vi "ImportCSV.vi"(8 "error in (no error)":errorcluster, 10 "selected path":path, 11 "Node Ref In":T1 format="%.0x") -> (0 "error out":errorcluster)   [LabVIEW 2024, in "Embedded TDMS Logger System Explorer.lvlib"]
doc: "Import the configuration of the Custom Device based on a CSV file. Note: Is legacy code and only maintained for the purposes of non-code users in a specific project set."
uses:
  Embedded TDMS Logger System Explorer.lvlib
  <vilib>/NI VeriStand/Custom Device API/Custom Device Item Ref.ctl
  Shared/File Classes/Meta Data.ctl
  <vilib>/NI VeriStand/Custom Device API/Custom Device Channel.ctl
  <vilib>/NI VeriStand/Custom Device API/Custom Device Channel Type.ctl
  <vilib>/Utility/file.llb/Read Delimited Spreadsheet (string).vi
  Shared/Constants.vi
  <vilib>/NI VeriStand/Custom Device API/Set Item Property (Boolean).vi
  <vilib>/NI VeriStand/Custom Device API/Set Item Property (Variant).vi
  <vilib>/NI VeriStand/Custom Device API/Set Item Property (I32).vi
  <vilib>/NI VeriStand/Custom Device API/Set Item Property (Dependent Node Pointer).vi
  <vilib>/Utility/file.llb/Write Delimited Spreadsheet (string).vi
  NationalInstruments.VeriStand.SystemStorage
  NationalInstruments.VeriStand.SystemDefinitionAPI
  <vilib>/NI VeriStand/Custom Device API/Custom Device API.lvlib
  Shared/Embedded TDMS Logger Shared.lvlib
  <vilib>/NI VeriStand/Custom Device Tools/Custom Device Utility Library/Custom Device Utility Library.lvlib
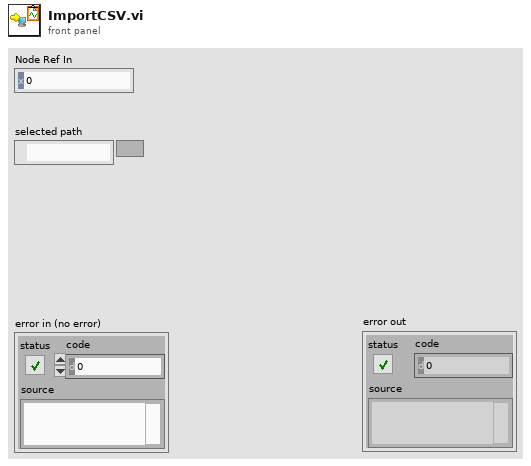
[diagram p1: front panel]
types:
  T1 = typedef "Custom Device API.lvlib/Custom Device Item Ref.ctl" = u64
  T2 = typedef "Custom Device API.lvlib/Custom Device Pointer.ctl" = refnum<k24>
  T3 = typedef "Custom Device API.lvlib/Custom Device Channel.ctl" = cluster{"Type":T4, "Units":string, "Default Value":dbl, "Faultable":bool, "Scalable":bool}
  T4 = typedef "Custom Device API.lvlib/Custom Device Channel Type.ctl" = enum16{"Input", "Output"}
  T5 = typedef "Meta Data.ctl" = cluster{"Key":string, "Value":string}
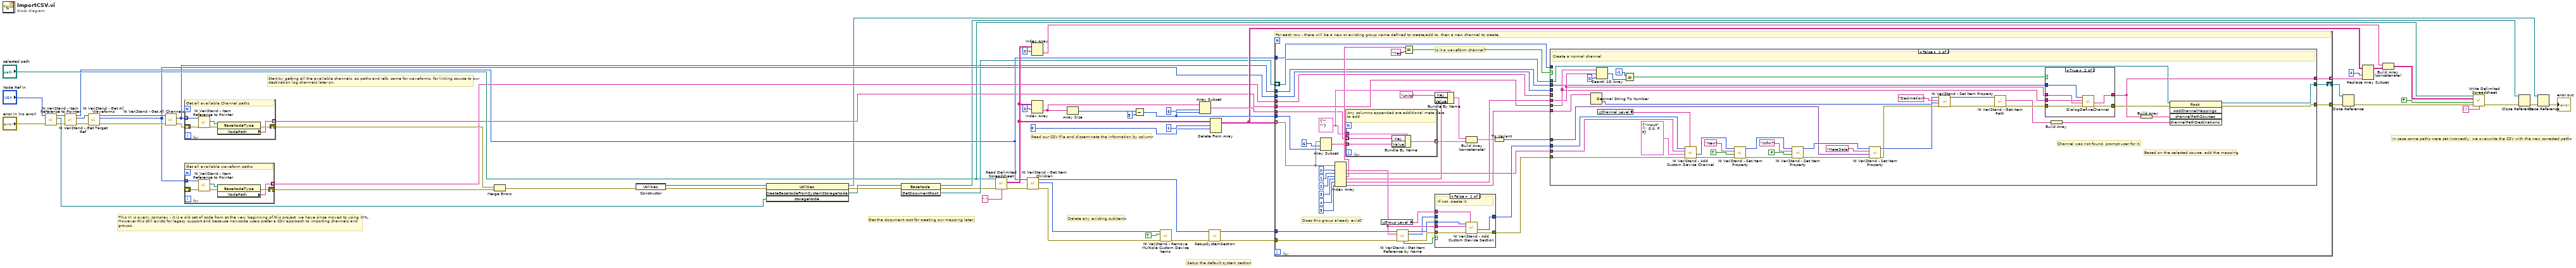
[diagram p0: block diagram]
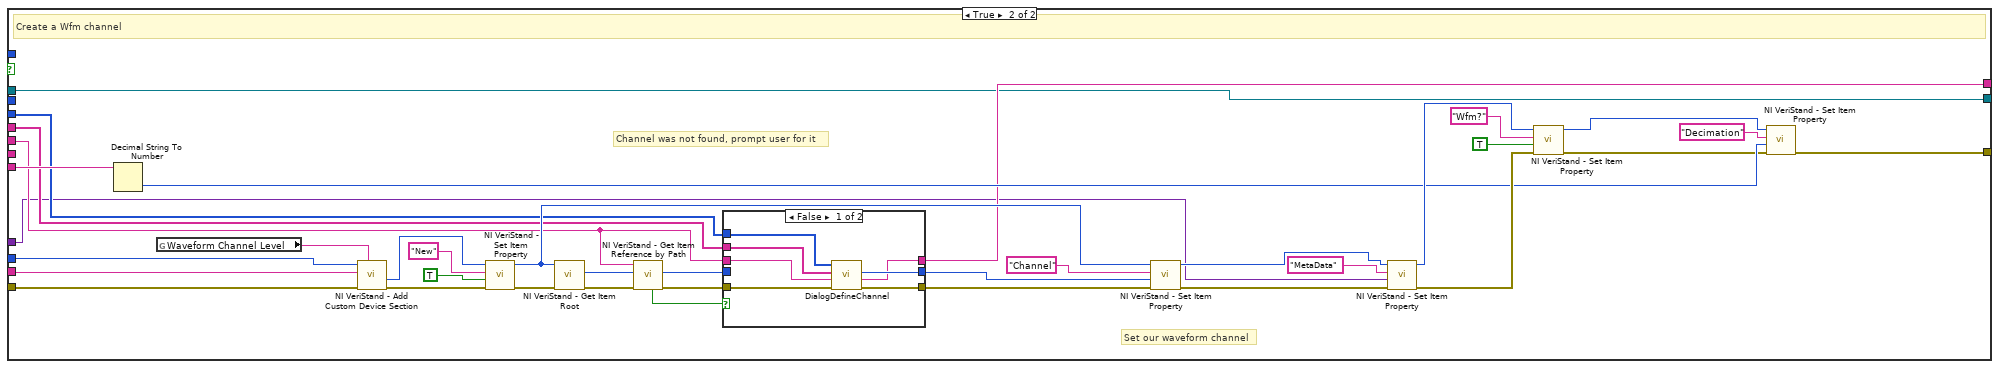
[diagram p3: hidden frame]
diagram:
  # "In case some paths were set incorrectly, we overwrite the CSV with the new corrected paths"
  # "Delete any existing subitems"
  # "Setup the default system section"
  # "Read our CSV file and disseminate the information by column"
  # "Get the document root for creating our mapping later."
  # "Start by getting all the available channels, as paths and refs, same for waveforms, for linking source to our\ndestination log channels later on."
  # "This VI is overly complex - it is a old set of code from at the very beginning of this project, we have since moved to using XML.\nHowever this still exists for legacy support and because non-code users prefer a CSV approach to importing channels and\ngroups."
  n1 = call <vilib>:"NI VeriStand - Item Reference to Pointer.vi"("error in (no error)"="error in (no error)", "Item Ref in"="Node Ref In") -> ("error out"=w18:errorcluster, "Node Pointer"=w23:T2, "Item Ref out"=w17:T1)  [unwired: 6 in, 1 out]
  n2 = call <vilib>:"NI VeriStand - Get Target Ref.vi"("error in"=w18, "Item Ref in"=w17) -> ("error out"=w19:errorcluster, "Target Ref"=w20:T1, "Item Ref out"=w16:T1)  [unwired: 6 in, 1 out]
  n3 = call <vilib>:"NI VeriStand - Get All Waveforms.vi"("error in"=w19, "Section Ref in"=w20) -> ("error out"=w27:errorcluster, "Waveform Refs"=w13:T1[], "Section Ref out"=w28:T1)  [unwired: 6 in, 1 out]
  n4 = call <vilib>:"NI VeriStand - Get All Channels.vi"("error in"=w27, "Section Ref in"=w28) -> ("error out"=w26:errorcluster, "Channel Refs"=w15:T1[])  [unwired: 6 in, 2 out]
  n5 = for {
    tunnel: w15 -> [w67] mode=indexing
    shift-right: [w62] -> w25
    shift-left: w26 -> [w66]
    tunnel: [w63] -> w14 mode=indexing
    # "Get all available Channel paths"
    n6 = call <vilib>:"NI VeriStand - Item Reference to Pointer.vi"("error in (no error)"=w66, "Item Ref in"=w67) -> ("error out"=w65:errorcluster, "Node Pointer"=w64:T2)  [unwired: 6 in, 2 out]
    n7 = property class="BaseNodeType"(reference=w64, error in=w65) -> (error out=w62:errorcluster, "NodePath"=w63:string)  [unwired: 1 out]
  }
  n8 = for {
    tunnel: w13 -> [w71] mode=indexing
    shift-right: [w69] -> w12
    shift-left: _ -> [w70]
    tunnel: [w68] -> w11 mode=indexing
    # "Get all available waveform paths"
    n9 = call <vilib>:"NI VeriStand - Item Reference to Pointer.vi"("error in (no error)"=w70, "Item Ref in"=w71) -> ("error out"=w73:errorcluster, "Node Pointer"=w72:T2)  [unwired: 6 in, 2 out]
    n10 = property class="BaseNodeType"(reference=w72, error in=w73) -> (error out=w69:errorcluster, "NodePath"=w68:string)  [unwired: 1 out]
  }
  n11 = Merge Errors(w25, w12) -> (w24:errorcluster)
  n12 = constructor class="Utilities"(error in=w24) -> (reference out=w32:refnum<k24>, error out=w31:errorcluster)  [unwired: 2 in, 1 out]
  n13 = invoke class="Utilities" method="CreateBaseNodeFromSystemStorageNode"(reference=w32, error in=w31, "storageNode"=w23) -> (reference out=w4:refnum<k24>, error out=w29:errorcluster, "CreateBaseNodeFromSystemStorageNode"=w30:refnum<k24>)  [unwired: 1 in, 1 out]
  n14 = invoke class="BaseNode" method="GetDocumentRoot"(reference=w30, error in=w29) -> (reference out=w5:refnum<k24>, error out=w9:errorcluster, "GetDocumentRoot"=w10:refnum<k24>)  [unwired: 1 in]
  n15 = call-poly <vilib>:"Read Delimited Spreadsheet.vi"("file path (dialog if empty)"="selected path", "error in (no error)"=w9, "delimiter (\\t)"="," ("delimiter (\\t)")) -> ("all rows"=w59:string[][], "error out"=w34:errorcluster)  [unwired: 7 in, 4 out]
  n16 = call <vilib>:"NI VeriStand - Get Item Children.vi"("error in (no error)"=w34, "Item Ref in"=w16) -> ("error out"=w2:errorcluster, "Child Refs"=w3:T1[], "Item Ref out"=w44:T1)  [unwired: 6 in, 1 out]
  n17 = Index Array(array=w59, index (row)=0) -> (element=w49:string[])  [unwired: 1 in]
  n18 = Index Array(array=w59, index (row)=0) -> (element=w55:string[])  [unwired: 1 in]
  n19 = Array Size(array=w55) -> (size(s)=w56:i32)
  n20 = Subtract(x=w56, y=5) -> (x-y=w61:i32)
  n21 = call <vilib>:"NI VeriStand - Remove Multiple Custom Device Items.vi"("error in (no error)"=w2, "Force Delete (F)"=TRUE, "Item Refs in"=w3) -> ("error out"=w45:errorcluster)  [unwired: 7 in, 1 out]
  n22 = Array Subset(array=w55, index=6, length=w61) -> (w60:string[])
  n23 = call "SetupSystemSection.vi"("error in (no error)"=w45, "Node Ptr"=w44) -> ("error out"=w46:errorcluster, "Parent Ref Out"=w47:T1)  [unwired: 4 in, 4 out]
  n24 = Delete From Array(array=w59, length=1, index (row)=0) -> (array with subset deleted=w53:string[][])  [unwired: 1 in, 1 out]
  n25 = for {
    tunnel: w53 -> [w79] mode=indexing
    tunnel: w47 -> [w110]
    tunnel: w16 -> [w95]
    tunnel: w46 -> [w94]
    tunnel: w13 -> [w92]
    tunnel: w11 -> [w91]
    tunnel: w14 -> [w90]
    tunnel: w15 -> [w93]
    tunnel: [w89] -> w38 mode=indexing
    tunnel: [w88] -> w41
    shift-right: [w87] -> w42
    shift-left: w10 -> [w86]
    tunnel: w60 -> [w75]
    tunnel: w61 -> [w78]
    w76 = T5 {"Key"="", "Value"=""} ("Meta Data")
    # "Does this group already exist?"
    # "Is it a waveform channel?"
    # "For each row - there will be a new or existing group name defined to create/add to, then a new channel to create."
    n26 = Array Subset(array=w79, index=6, length=w78) -> (w77:string[])
    n27 = Index Array(array=w79, index #1=0 ("index"), index #2=1 ("index"), index #3=2 ("index"), index #4=3 ("index"), index #5=4 ("index"), index #6=5 ("index")) -> (element #1=w107:string, element #2=w99:string, element #3=w103:string, element #4=w83:string, element #5=w97:string, element #6=w96:string)
    n28 = for {
      tunnel: w77 -> [w118] mode=indexing
      tunnel: w76 -> [w120]
      tunnel: w75 -> [w119] mode=indexing
      tunnel: [w117] -> w74 mode=indexing
      # "Any columns appended are additional meta data to add"
      n29 = Bundle By Name(cluster=w120, "Key"=w119, "Value"=w118) -> (w117:T5)
    }
    n30 = global read "Constants.vi" "Group Level"() -> (w104:string)
    n31 = call <vilib>:"NI VeriStand - Get Item Reference by Name.vi"("error in (no error)"=w94, "Item Name"=w107, "Parent Ref in"=w110) -> ("error out"=w106:errorcluster, "Item Ref"=w105:T1, "Parent Ref out"=w108:T1, "Found"=w109:bool)  [unwired: 5 in]
    n32 = Equal?(x=w103, y="Yes") -> (x = y?=w101:bool)
    n33 = Bundle By Name(cluster=w76, "Key"="Units", "Value"=w83) -> (w80:T5)
    n34 = case shown="False" w109 {
      tunnel: w108 -> [w221 _]
      tunnel: w107 -> [w220 _]
      tunnel: w106 -> [w219 w222]
      tunnel: [w218 w223] -> w100
      tunnel: w105 -> [_ w223]
      tunnel: [w217 w222] -> w98
      tunnel: w104 -> [w216 _]
      frame False {
        # "If not, create it"
        n35 = call <vilib>:"NI VeriStand - Add Custom Device Section.vi"("GUID (Default Section)"=w216, "error in (no error)"=w219, "Section Name"=w220, "Parent Ref in"=w221) -> ("error out"=w217:errorcluster, "Section Ptr"=w218:T1)  [unwired: 4 in, 2 out]
      }
      frame True {
      }
    }
    n36 = Build Array (concatenate)(w80, w74) -> (w82:T5[])
    n37 = To Variant(anything=w82) -> (Variant=w81:variant)
    n38 = case shown="False" w101 {
      tunnel: w100 -> [w148 w193]
      tunnel: w99 -> [w145 w191]
      tunnel: w98 -> [w147 w190]
      tunnel: w97 -> [w130 w179]
      tunnel: w96 -> [w142 w189]
      tunnel: w95 -> [_ _]
      tunnel: w86 -> [w135 w170]
      tunnel: w93 -> [w127 _]
      tunnel: w92 -> [_ w178]
      tunnel: w91 -> [_ w177]
      tunnel: w90 -> [w128 _]
      tunnel: [w125 w172] -> w89
      tunnel: [w123 w171] -> w88
      tunnel: [w122 w170] -> w87
      tunnel: w81 -> [w121 w169]
      frame False {
        # "Channel was not found, prompt user for it."
        # "Based on the selected source, add the mapping"
        # "Create a normal channel"
        n39 = Decimal String To Number(string=w142) -> (number=w143:i32)  [unwired: 2 in, 1 out]
        n40 = Search 1D Array(1D array=w128, element=w130, start index (0)=0) -> (index of element=w133:i32)
        n41 = global read "Constants.vi" "Channel Level"() -> (w146:string)
        n42 = Equal?(x=-1, y=w133) -> (x = y?=w131:bool)
        n43 = call <vilib>:"NI VeriStand - Add Custom Device Channel.vi"("GUID (Default Channel)"=w146, "error in (no error)"=w147, "Channel"=T3 {"Type"=enum."Input", "Units"="", "Default Value"=0.0, "Faultable"=FALSE, "Scalable"=FALSE}, "Channel Name"=w145, "Parent Ref in"=w148) -> ("error out"=w155:errorcluster, "Channel Ref"=w156:T1)  [unwired: 3 in, 2 out]
        n44 = call-poly <vilib>:"NI VeriStand - Set Item Property.vi"("error in (no error)"=w155, "Value"=TRUE, "Property Name"="New", "Item Ref in"=w156) -> ("error out"=w158:errorcluster, "Item Ref out"=w157:T1)  [unwired: 5 in, 1 out]
        n45 = call-poly <vilib>:"NI VeriStand - Set Item Property.vi"("error in (no error)"=w158, "Value"=FALSE, "Property Name"="Wfm?", "Item Ref in"=w157) -> ("error out"=w160:errorcluster, "Item Ref out"=w159:T1)  [unwired: 5 in, 1 out]
        n46 = call-poly <vilib>:"NI VeriStand - Set Item Property.vi"("error in (no error)"=w160, "Value"=w121, "Property Name"="MetaData", "Item Ref in"=w159) -> ("error out"=w140:errorcluster, "Item Ref out"=w141:T1)  [unwired: 5 in, 1 out]
        n47 = call-poly <vilib>:"NI VeriStand - Set Item Property.vi"("error in (no error)"=w140, "Value"=w143, "Property Name"="Decimation", "Item Ref in"=w141) -> ("error out"=w136:errorcluster, "Item Ref out"=w137:T1)  [unwired: 5 in, 1 out]
        n48 = call <vilib>:"NI VeriStand - Get Item Path.vi"("error in (no error)"=w136, "Item Ref in"=w137) -> ("error out"=w126:errorcluster, "Path"=w124:string)  [unwired: 6 in, 2 out]
        n49 = case shown="True" w131 {
          tunnel: [w162 w168] -> w125
          tunnel: w130 -> [w162 w165]
          tunnel: [w161 w167] -> w129
          tunnel: w128 -> [_ w166]
          tunnel: w127 -> [_ w164]
          tunnel: w126 -> [w161 w163]
          frame False {
          }
          frame True {
            n50 = call "DialogDefineChannel.vi"("error in"=w163, "Input String"=w165, "Available Paths"=w166, "Available Refs"=w164) -> ("error out"=w167:errorcluster, "Selected Path"=w168:string)  [unwired: 4 in, 2 out]
          }
        }
        n51 = Build Array(w124) -> (w138:string[])
        n52 = Build Array(w125) -> (w139:string[])
        n53 = invoke class="Root" method="AddChannelMappings"(reference=w135, error in=w129, "channelPathSources"=w139, "channelPathDestinations"=w138) -> (reference out=w122:refnum<k24>, error out=w123:errorcluster)  [unwired: 1 in, 3 out]
      }
      frame True {
        # "Set our waveform channel"
        # "Channel was not found, prompt user for it"
        # "Create a Wfm channel"
        n54 = Decimal String To Number(string=w189) -> (number=w183:i32)  [unwired: 2 in, 1 out]
        n55 = global read "Constants.vi" "Waveform Channel Level"() -> (w192:string)
        n56 = call <vilib>:"NI VeriStand - Add Custom Device Section.vi"("GUID (Default Section)"=w192, "error in (no error)"=w190, "Section Name"=w191, "Parent Ref in"=w193) -> ("error out"=w200:errorcluster, "Section Ptr"=w201:T1)  [unwired: 3 in, 3 out]
        n57 = call-poly <vilib>:"NI VeriStand - Set Item Property.vi"("error in (no error)"=w200, "Value"=TRUE, "Property Name"="New", "Item Ref in"=w201) -> ("error out"=w186:errorcluster, "Item Ref out"=w187:T1)  [unwired: 5 in, 1 out]
        n58 = call <vilib>:"NI VeriStand - Get Item Root.vi"("error in (no error)"=w186, "Item Ref in"=w187) -> ("error out"=w185:errorcluster, "Root Ref out"=w188:T1)  [unwired: 6 in, 2 out]
        n59 = call <vilib>:"NI VeriStand - Get Item Reference by Path.vi"("error in (no error)"=w185, "Root Ref"=w188, "Item Path in"=w179) -> ("error out"=w176:errorcluster, "Item Ref"=w173:T1, "Found"=w184:bool)  [unwired: 5 in, 1 out]
        n60 = case shown="False" w184 {
          tunnel: w179 -> [w212 w213]
          tunnel: w178 -> [w210 _]
          tunnel: w177 -> [w211 _]
          tunnel: w176 -> [w207 w214]
          tunnel: [w208 w214] -> w175
          tunnel: [w209 w215] -> w174
          tunnel: w173 -> [_ w215]
          tunnel: [w206 w213] -> w172
          frame False {
            n61 = call "DialogDefineChannel.vi"("error in"=w207, "Input String"=w212, "Available Paths"=w211, "Available Refs"=w210) -> ("error out"=w208:errorcluster, "Selected Path"=w206:string, "Selected Ref"=w209:T1)  [unwired: 4 in, 1 out]
          }
          frame True {
          }
        }
        n62 = call-poly <vilib>:"NI VeriStand - Set Item Property.vi"("error in (no error)"=w175, "Dependent Node Ref"=w174, "Property Name"="Channel", "Item Ref in"=w187) -> ("error out"=w202:errorcluster, "Item Ref out"=w203:T1)  [unwired: 5 in, 1 out]
        n63 = call-poly <vilib>:"NI VeriStand - Set Item Property.vi"("error in (no error)"=w202, "Value"=w169, "Property Name"="MetaData", "Item Ref in"=w203) -> ("error out"=w205:errorcluster, "Item Ref out"=w204:T1)  [unwired: 5 in, 1 out]
        n64 = call-poly <vilib>:"NI VeriStand - Set Item Property.vi"("error in (no error)"=w205, "Value"=TRUE, "Property Name"="Wfm?", "Item Ref in"=w204) -> ("error out"=w180:errorcluster, "Item Ref out"=w182:T1)  [unwired: 5 in, 1 out]
        n65 = call-poly <vilib>:"NI VeriStand - Set Item Property.vi"("error in (no error)"=w180, "Value"=w183, "Property Name"="Decimation", "Item Ref in"=w182) -> ("error out"=w171:errorcluster)  [unwired: 5 in, 2 out]
      }
    }
  }
  n66 = Close Reference(reference=w42, error in (no error)=w41) -> (error out=w33:errorcluster)
  n67 = Replace Array Subset(array=w53, new element=w38, index (col)=4 ("index")) -> (w51:string[][])  [unwired: 1 in]
  n68 = Build Array (concatenate)(w49, w51) -> (w50:string[][])
  n69 = call-poly <vilib>:"Write Delimited Spreadsheet.vi"("file path (dialog if empty)"="selected path", "2D data"=w50, "append to file? (new file:F)"=FALSE, "error in (no error)"=w33, "delimiter (\\t)"="," ("delimiter (\\t)")) -> ("error out"=w6:errorcluster)  [unwired: 9 in, 1 out]
  n70 = Close Reference(reference=w5, error in (no error)=w6) -> (error out=w8:errorcluster)
  n71 = Close Reference(reference=w4, error in (no error)=w8) -> (error out=→"error out":errorcluster)
